vi "Desentramador_Serial_Array.vi"(0 "Trama_Serial":string, 1 "Separador":string) -> (5 "array":dbl[](array[numeric]))   [LabVIEW 2019]
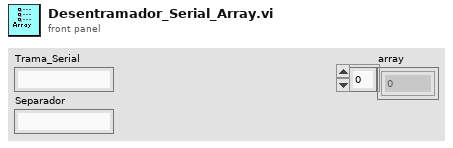
[diagram p1: front panel]
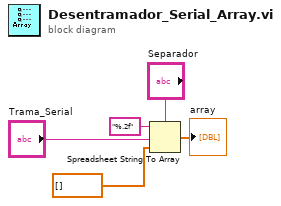
[diagram p0: block diagram]
diagram:
  n1 = Spreadsheet String To Array(delimiter (Tab)="Separador", format string="%.2f", spreadsheet string="Trama_Serial", array type (2D Dbl)=dbl[] []) -> (array=→"array":dbl[])
